vi "SortArray_H_to_L.vi"() -> ()   [LabVIEW 2011]
panel:
  out "mu08ArrayOut":u8[](array[numeric])
  out "mu08ArrayOutIndexCount":u8
  out "mu08Max":u8
  out "mu08Temp":u8
  in  "ArrayInput":u8[](array[numeric])
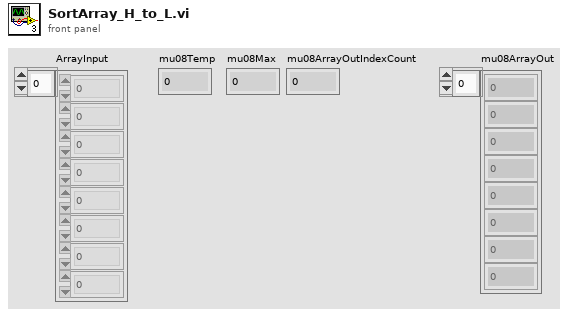
[diagram p1: front panel]
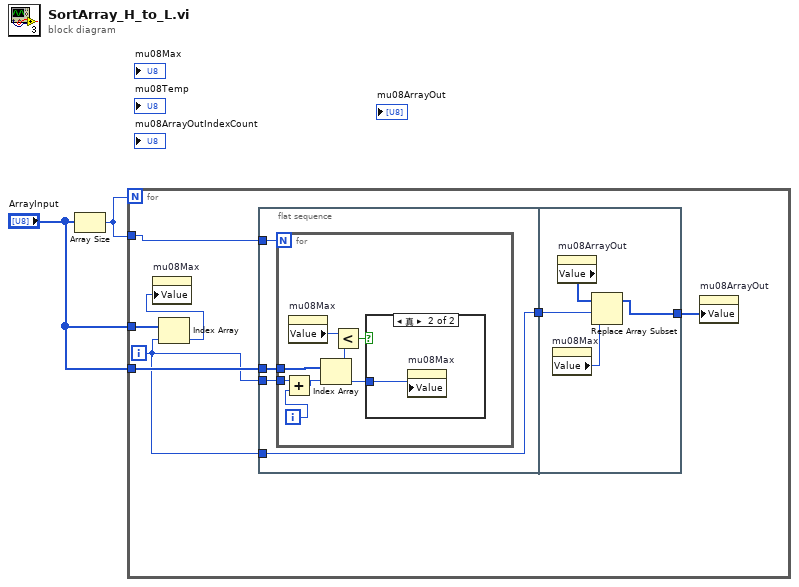
[diagram p0: block diagram]
diagram:
  n1 = Array Size(array="ArrayInput") -> (size(s)=w2:i32)
  n2 = for {
    N: w2 -> [_]
    tunnel: "ArrayInput" -> [w9]
    tunnel: w2 -> [w4]
    tunnel: "ArrayInput" -> [w7]
    i -> [w3]
    n3 = Index Array(array=w9, index=w3) -> (element=w8:u8)
    n4 = property on="mu08Max" class="DigNum (严格)"("Value"=w8) -> ()  [unwired: 2 in, 2 out]
    n5 = flat-sequence {
      tunnel: w7 -> [w13]
      tunnel: w3 -> [w12]
      tunnel: [w12] -> w6
      tunnel: w4 -> [w11]
      tunnel: w3 -> [w10]
      tunnel: w6 -> [w24]
      tunnel: [w22] -> w5
      frame #0 {
        n6 = for {
          N: w11 -> [_]
          tunnel: w13 -> [w20]
          tunnel: w10 -> [w15]
          i -> [w16]
          n7 = Add(x=w15, y=w16) -> (x+y=w14:i32)
          n8 = property on="mu08Max" class="DigNum (严格)"() -> ("Value"=w19:u8)  [unwired: 2 in, 2 out]
          n9 = Index Array(array=w20, index=w14) -> (element=w17:u8)
          n10 = Less?(x=w19, y=w17) -> (x < y?=w18:bool)
          n11 = case shown="真" w18 {
            tunnel: w17 -> [_ w21]
            frame False {
            }
            frame True {
              n12 = property on="mu08Max" class="DigNum (严格)"("Value"=w21) -> ()  [unwired: 2 in, 2 out]
            }
          }
        }
      }
      frame #1 {
        n13 = property on="mu08Max" class="DigNum (严格)"() -> ("Value"=w23:u8)  [unwired: 2 in, 2 out]
        n14 = property on="mu08ArrayOut" class="Arr (严格)"() -> ("Value"=w25:u8[])  [unwired: 2 in, 2 out]
        n15 = Replace Array Subset(array=w25, new element=w23, index=w24) -> (w22:u8[])
      }
    }
    n16 = property on="mu08ArrayOut" class="Arr (严格)"("Value"=w5) -> ()  [unwired: 2 in, 2 out]
  }
